vi "Configure NPLC.vi"(6 "Power Line Cycle (1)":dbl=1.0, 8 "error in (no error)":errorcluster, 9 "Channel List(\"\")":string, 10 "Function (0: Voltage DC)":i32(ring) items=[" Voltage DC"=0, "Current DC"=2, "Resistance"=4, "4-wire Resistance"=5, "Diode"=6, "Temperature"=8, "Voltage Ratio"=12], 11 "VISA resource name":refnum<visa-resource-name>) -> (0 "error out":errorcluster, 3 "VISA resource name out":refnum<visa-resource-name>)   [LabVIEW 2016, in "Keithley DMM6500 DAQ6500 Series.lvlib"]
doc: "Configures number of power line cycle."
uses:
  Keithley DMM6500 DAQ6500 Series.lvlib
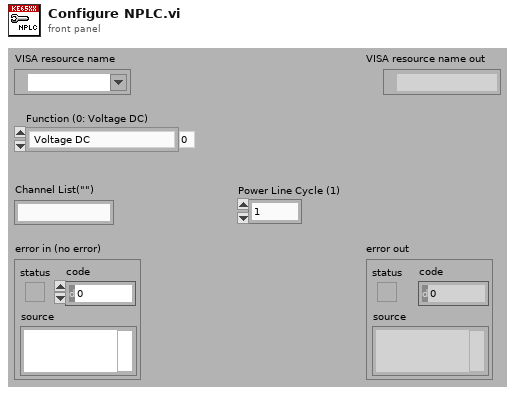
[diagram p1: front panel]
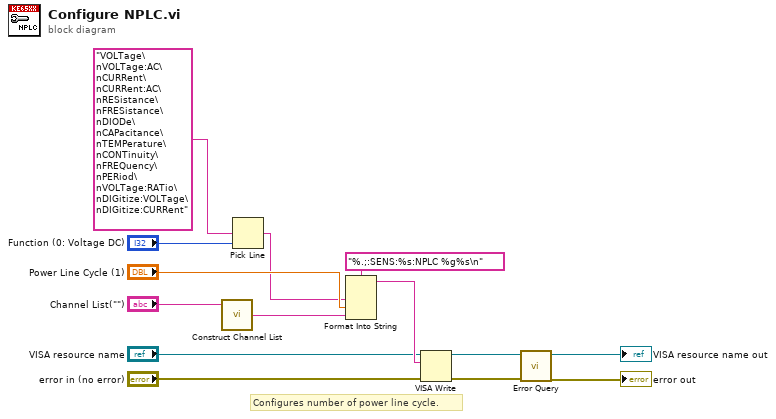
[diagram p0: block diagram]
diagram:
  # "Configures number of power line cycle."
  n1 = call "Construct Channel List.vi"("Channel List"="Channel List(\"\")") -> ("Channel List String"=w2:string)  [unwired: 2 in]
  n2 = Pick Line(multi-line string="VOLTage\nVOLTage:AC\nCURRent\nCURRent:AC\nRESistance\nFRESistance\nDIODe\nCAPacitance\nTEMPerature\nCONTinuity\nFREQuency\nPERiod\nVOLTage:RATio\nDIGitize:VOLTage\nDIGitize:CURRent", line index="Function (0: Voltage DC)") -> (output string=w5:string)  [unwired: 1 in]
  n3 = Format Into String(format string="%.;:SENS:%s:NPLC %g%s\n", w5, "Power Line Cycle (1)", w2) -> (resulting string=w12:string)  [unwired: 2 in, 1 out]
  n4 = VISA Write(VISA resource name="VISA resource name", write buffer=w12, error in (no error)="error in (no error)") -> (VISA resource name out=w9:refnum<visa-resource-name>, error out=w8:errorcluster)  [unwired: 1 out]
  n5 = call "Error Query.vi"("error in (no error)"=w8, "VISA resource name"=w9) -> ("error out"=→"error out":errorcluster, "VISA resource name out"=→"VISA resource name out":refnum<visa-resource-name>)  [unwired: 6 in, 2 out]
